vi "VIQA Update MCLB.vi"(8 "error in (no error)":errorcluster, 9 "Reset TopLeft? (F)":bool, 10 "Items":T1[](array[typedef]), 11 "MCLB":refnum<vi>) -> (0 "error out":errorcluster, 3 "dup MCLB":refnum<vi>)   [LabVIEW 2018, in "VI Quality.lvlib"]
uses:
  VI Quality.lvlib
  <vilib>/Utility/miscctls.llb/LVRowAndColumnUnsignedTypeDef.ctl
  Controls/VIQA Audit.ctl
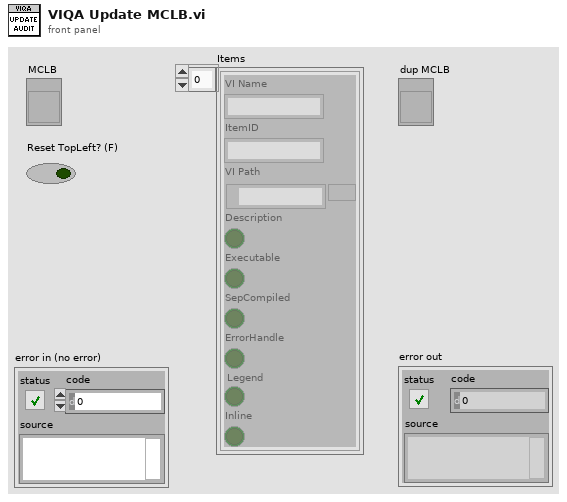
[diagram p1: front panel]
types:
  T1 = typedef "VI Quality.lvlib/VIQA Audit.ctl" = cluster{"VI Name":string, "ItemID":string, "VI Path":path, "Description":bool, "Executable":bool, "SepCompiled":bool, "ErrorHandle":bool, "Legend":bool, "Inline":bool}
  T2 = typedef "LVRowAndColumnUnsignedTypeDef.ctl" = cluster{"Row":u32, "Column":u32}
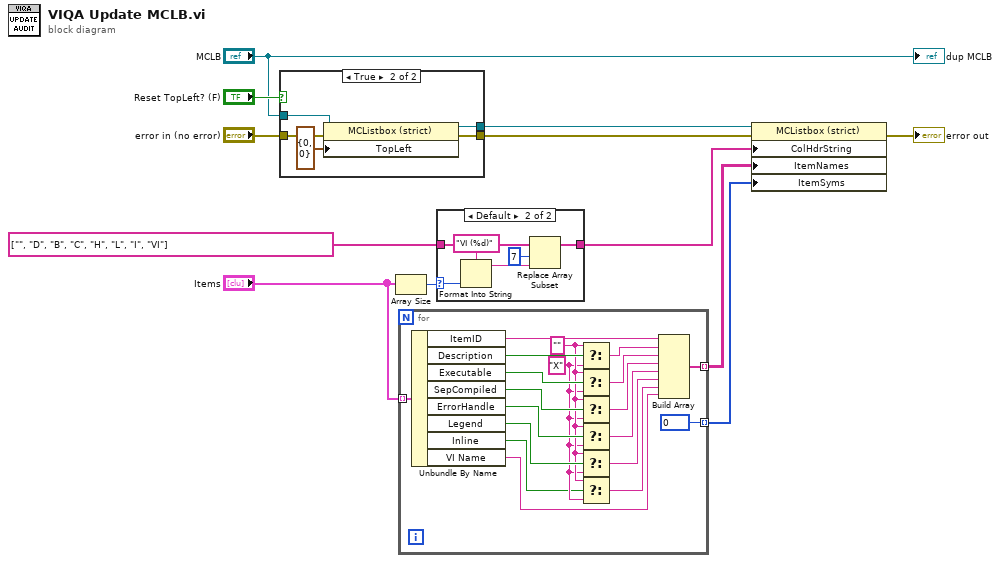
[diagram p0: block diagram]
diagram:
  n1 = case shown="True" "Reset TopLeft? (F)" {
    tunnel: "error in (no error)" -> [w14 w19]
    tunnel: [w14 w18] -> w6
    tunnel: "MCLB" -> [w13 w17]
    tunnel: [w13 w16] -> w5
    frame False {
    }
    frame True {
      n2 = property class="MCListbox (strict)"(reference=w17, error in=w19, "TopLeft"=T2 {"Row"=0, "Column"=0} ("Top Left Visible Cell")) -> (reference out=w16:refnum<vi>, error out=w18:errorcluster)
    }
  }
  n3 = Array Size(array="Items") -> (size(s)=w3:i32)
  n4 = for {
    tunnel: "Items" -> [w38] mode=indexing
    tunnel: [w32] -> w10 mode=indexing
    tunnel: [0] -> w1 mode=indexing
    w24 = "X" ("f")
    w25 = ""
    n5 = Unbundle By Name(w38) -> ("ItemID"=w21:string, "Description"=w37:bool, "Executable"=w36:bool, "SepCompiled"=w35:bool, "ErrorHandle"=w34:bool, "Legend"=w33:bool, "Inline"=w23:bool, "VI Name"=w26:string)
    n6 = Select(t=w25, s=w37, f=w24) -> (s? t:f=w31:string)
    n7 = Select(t=w25, s=w36, f=w24) -> (s? t:f=w30:string)
    n8 = Select(t=w25, s=w35, f=w24) -> (s? t:f=w29:string)
    n9 = Select(t=w25, s=w34, f=w24) -> (s? t:f=w28:string)
    n10 = Select(t=w25, s=w33, f=w24) -> (s? t:f=w27:string)
    n11 = Select(t=w25, s=w23, f=w24) -> (s? t:f=w22:string)
    n12 = Build Array(w21, w31, w30, w29, w28, w27, w22, w26) -> (w32:string[])
  }
  n13 = case shown="Default" w3 {
    selector: w3 -> [_ w40]
    tunnel: [w39 w45] -> w12
    tunnel: string[] ["", "D", "B", "C", "H", "L", "I", "VI"] ("Column Header Strings[]") -> [w39 w41]
    frame 0 {
    }
    frame Default {
      n14 = Format Into String(format string="VI (%d)", w40) -> (resulting string=w43:string)  [unwired: 2 in, 1 out]
      n15 = Replace Array Subset(array=w41, new element=w43, index=7) -> (w45:string[])
    }
  }
  n16 = property class="MCListbox (strict)"(reference=w5, error in=w6, "ColHdrString"=w12, "ItemNames"=w10, "ItemSyms"=w1) -> (error out=→"error out":errorcluster)  [unwired: 1 out]
  "dup MCLB" <- "MCLB"
